vi "总磷总氮通讯.vi"() -> ()   [LabVIEW 2016, in "斯坦道总磷总氮.lvlib"]
uses:
  <vilib>/NI/Modbus Library/API/Wrapper/Create TCP Slave.vi
  <vilib>/Utility/config.llb/Write Key (Boolean).vi
  <vilib>/Utility/config.llb/Write Key (String).vi
  <vilib>/Plasmionique/MB Master/MB_Master/MB_Master.lvclass
  <vilib>/NI/Modbus Library/API/slave/Modbus Slave.lvclass
  <vilib>/Utility/config.llb/NI_LVConfig.lvlib
  <vilib>/Plasmionique/MB Master/MB Master.lvlib
  <vilib>/NI/Modbus Library/API/Wrapper/API Main.lvlib
  <vilib>/ptbypt/NI_PtbyPt.lvlib
panel:
  out "氨氮状态告警区":u16[](array[numeric])
  out "氨氮测量数据区":u16[](array[numeric])
  out "COD测量数据区":u16[](array[numeric])
  out "COD状态告警区":u16[](array[numeric])
  out "总氮测量数据区":u16[](array[numeric])
  out "总氮状态告警区":u16[](array[numeric])
  out "总磷状态告警区":u16[](array[numeric])
  out "总磷测量数据区":u16[](array[numeric])
  out "序列号":string
  out "状态告警区":T1 {"告警代码" items=["无告警", "缺试剂告警", "缺水样告警", "缺蒸馏水告警", "缺标液告警", "仪表漏液告警", "标定异常告警", "超量程告警", "加热异常", "低试剂预警", "超上限告警", "超下限告警", "仪表内部其他异常", "滴定异常告警", "电极异常告警", "量程切换告警", "参数设置告警", "PH电极电位异常", "电导率电极异常", "浊度光度异常", "溶解氧电极异常", "溶解氧光强异常", "温度异常告警", "PH异常告警", "溶解氧异常告警", "电导率异常告警", "浊度异常告警", "叶绿素异常告警", "藻密度异常告警", "蓝绿藻异常告警", "ORP异常告警", "氨氮异常告警", "清洁刷异常告警", "SD卡异常告警", "蓝牙异常告警", "Wifi异常告警", "流程异常告警"]; "故障代码" items=["无故障", "电机故障", "温度故障", "通讯故障", "滴定故障"]}
  out "测量数据区":T2 {"单位" items=["ug/L", "mg/L", "ppm", "mg/m3", "cm", "ppb", "ug/m3", "%", "nmol/mol", "umol/mol", "MPN/L", "MPN/100ml", "ng/m3", "NTU", "无量纲", "ms/cm", "us/cm", "℃", "mV", "万个/L"]}
  out "status":bool
  out "关键参数区":T3
  in  "读关键参数区":bool
  in  "读状态告警区":bool
  in  "读测量数据区":bool
  in  "站号":u16(ring) items=["总磷"=1, "氨氮"=3]
  in  "停止":bool
  in  "启动":bool
  in  "控制命令":u16(ring) items=["启动测量"=1, "标样核查"=2, "零点核查"=3, "跨度核查"=4, "空白测试"=5, "平行样测试"=6, "加标回收"=7, "空白校准"=8, "标样校准"=9, "初始化（清洗）"=10, "停止测试"=11, "仪器重启"=12, "校时"=13, "模式设置"=14, "测量间隔设置"=15]
  in  "控制命令参数":u16[](array[numeric]) format="%04xH"
  in  "VISA Resource":refnum<visa-resource-name>
  in  "启用模块":bool
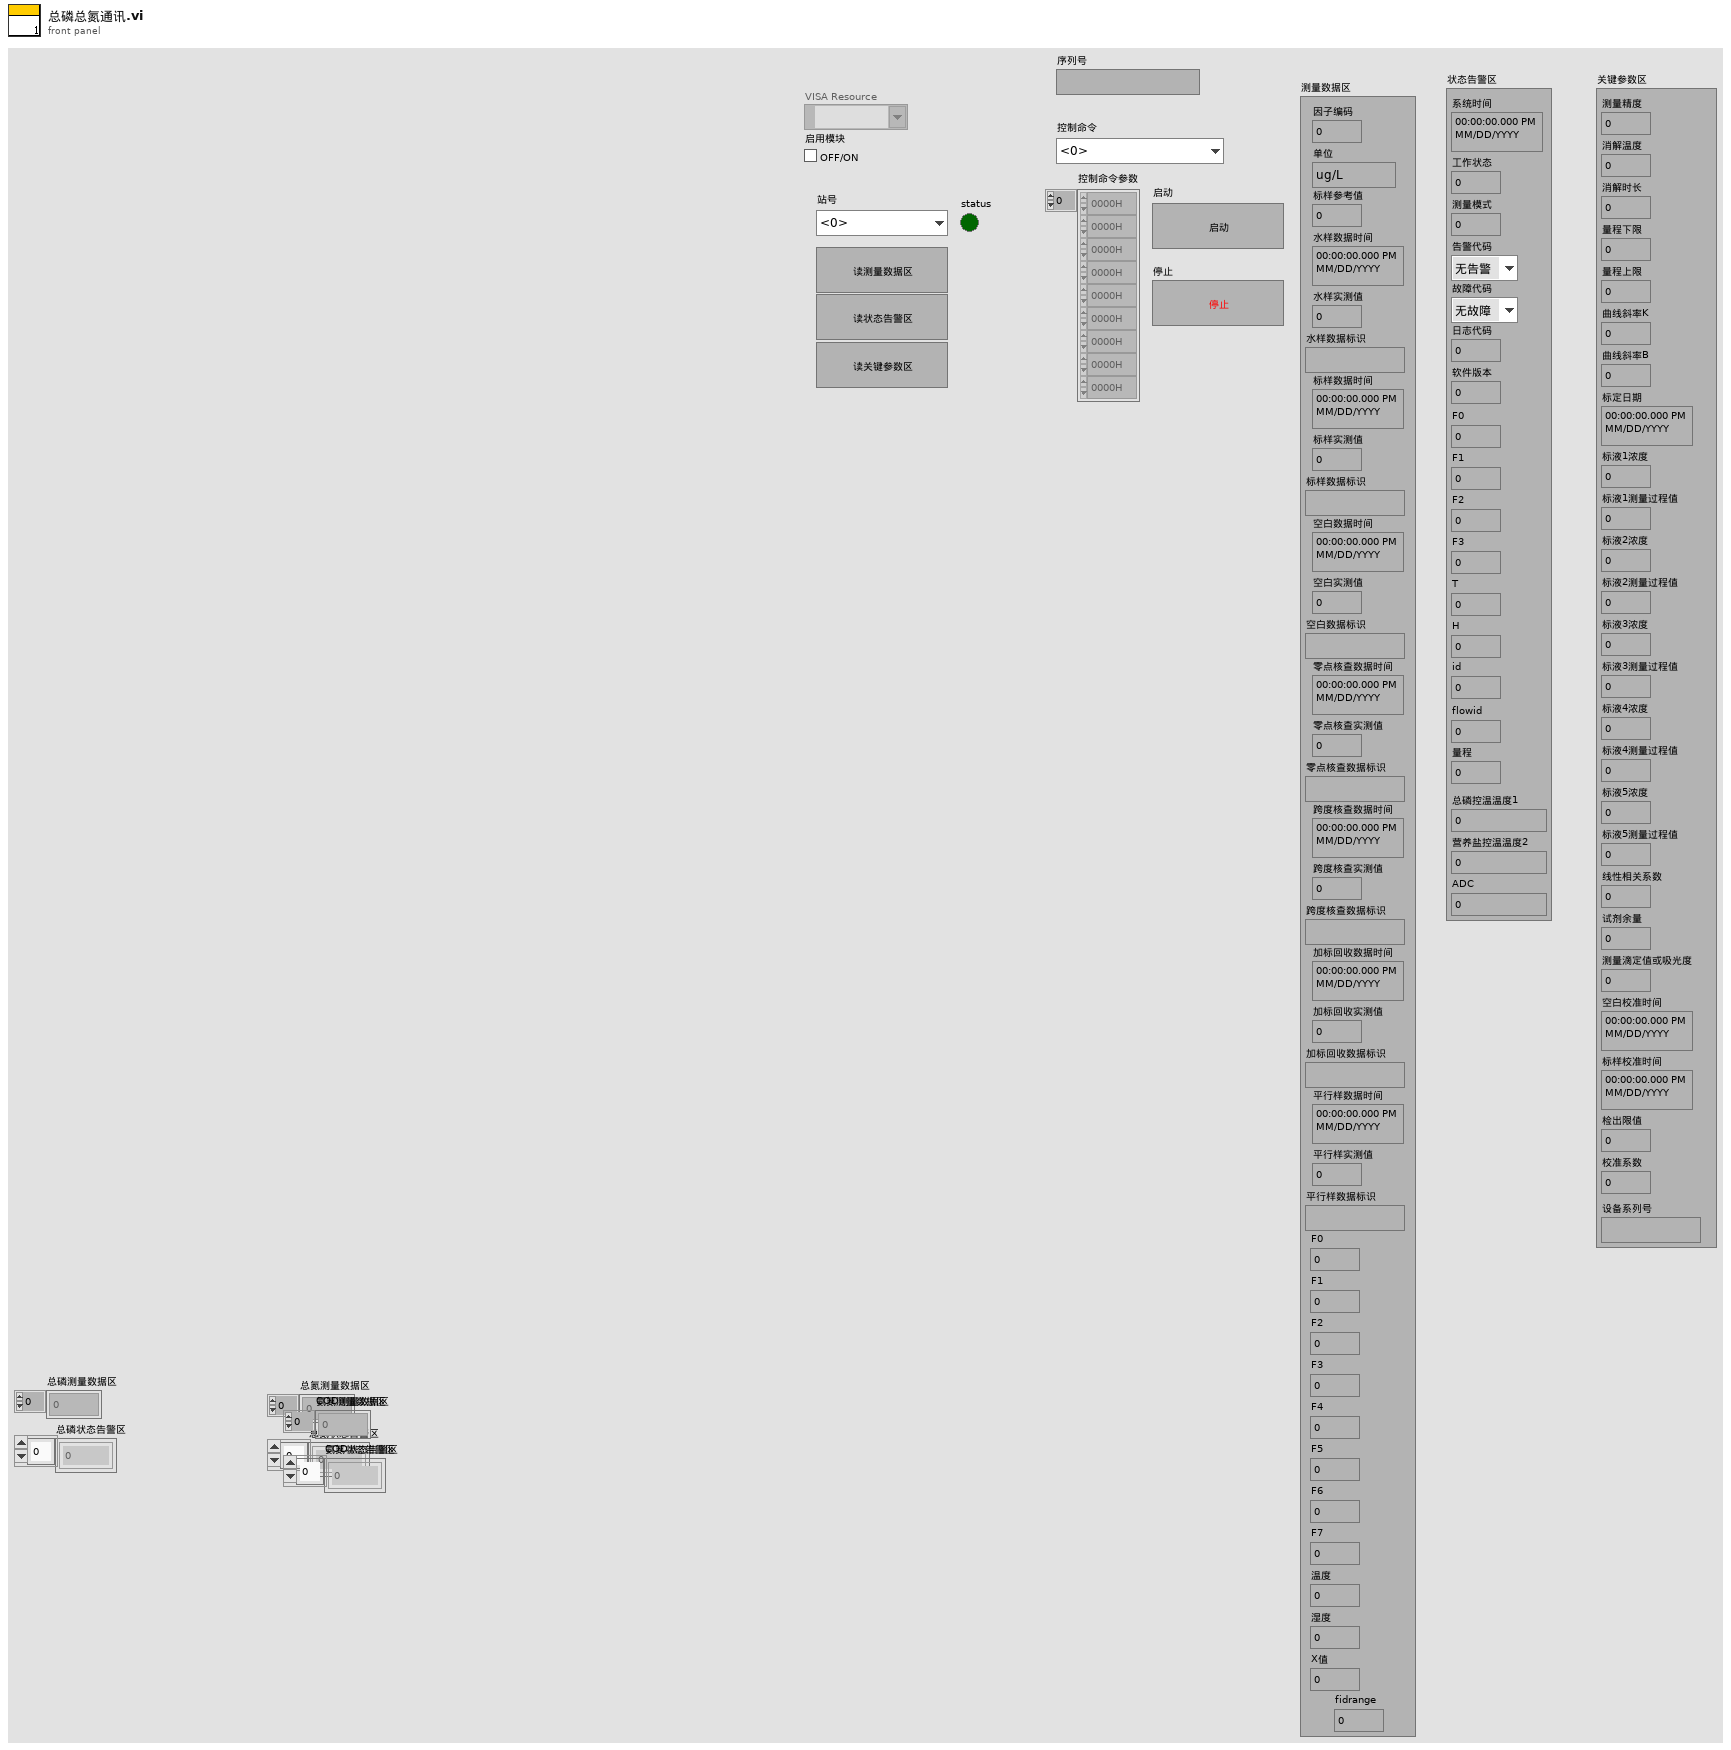
[diagram p1: front panel]
types:
  T1 = cluster{"系统时间":timestamp, "工作状态":u16, "测量模式":u16, "告警代码":u16, "故障代码":u16, "日志代码":u16, "软件版本":u16, "F0":sgl, "F1":sgl, "F2":sgl, "F3":sgl, "T":sgl, "H":sgl, "id":u16, "flowid":u16, "量程":u16, "总磷控温温度1":sgl, "营养盐控温温度2":sgl, "ADC":sgl}
  T2 = cluster{"因子编码":u32, "单位":u16, "标样参考值":sgl, "水样数据时间":timestamp, "水样实测值":sgl, "水样数据标识":string, "标样数据时间":timestamp, "标样实测值":sgl, "标样数据标识":string, "空白数据时间":timestamp, "空白实测值":sgl, "空白数据标识":string, "零点核查数据时间":timestamp, "零点核查实测值":sgl, "零点核查数据标识":string, "跨度核查数据时间":timestamp, "跨度核查实测值":sgl, "跨度核查数据标识":string, "加标回收数据时间":timestamp, "加标回收实测值":sgl, "加标回收数据标识":string, "平行样数据时间":timestamp, "平行样实测值":sgl, "平行样数据标识":string, "F0":sgl, "F1":sgl, "F2":sgl, "F3":sgl, "F4":sgl, "F5":sgl, "F6":sgl, "F7":sgl, "温度":sgl, "湿度":sgl, "X值":sgl, "fidrange":u16}
  T3 = cluster{"测量精度":u16, "消解温度":u16, "消解时长":u16, "量程下限":sgl, "量程上限":sgl, "曲线斜率K":sgl, "曲线斜率B":sgl, "标定日期":timestamp, "标液1浓度":sgl, "标液1测量过程值":sgl, "标液2浓度":sgl, "标液2测量过程值":sgl, "标液3浓度":sgl, "标液3测量过程值":sgl, "标液4浓度":sgl, "标液4测量过程值":sgl, "标液5浓度":sgl, "标液5测量过程值":sgl, "线性相关系数":sgl, "试剂余量":u32, "测量滴定值或吸光度":sgl, "空白校准时间":timestamp, "标样校准时间":timestamp, "检出限值":sgl, "校准系数":sgl, "设备系列号":string}
  T4 = cluster{"COD":bool, "氨氮":bool, "总氮":bool, "总磷":bool}
  T5 = typedef "NI_LVConfig.lvlib/Config Data RefNum.ctl" = refnum<k1>
  T6 = enum8{"Enabled", "Disabled", "Disabled and Grayed Out"}
  T7 = cluster{"时间标识":timestamp, "设备":string, "日志信息":string, "备注":string}
  T8 = cluster{"系统时间":timestamp, "工作状态":enum16{"空闲", "水样测试", "标样核查", "零点核查", "跨度核查", "空白测试", "平行样测试", "加标回收", "空白校准", "标样校准", "初始化（清洗）"}, "测量模式":enum16{"待机", "连续模式", "周期模式", "定点模式", "受控模式", "手动模式"}, "告警代码":u16, "故障代码":u16, "日志代码":u16, "软件版本":u16, "F0":sgl, "F1":sgl, "F2":sgl, "F3":sgl, "T":sgl, "H":sgl, "id":u16, "flowid":u16, "量程":u16, "总磷控温温度1":sgl, "营养盐控温温度2":sgl, "ADC":sgl}
  T9 = cluster{"水样测试量程模式":enum16{"H", "L", "AUTO"}, "空白核查量程模式":enum16{"H", "L", "AUTO"}, "跨度核查量程模式":enum16{"H", "L", "AUTO"}, "加标回收量程模式":enum16{"H", "L", "AUTO"}}
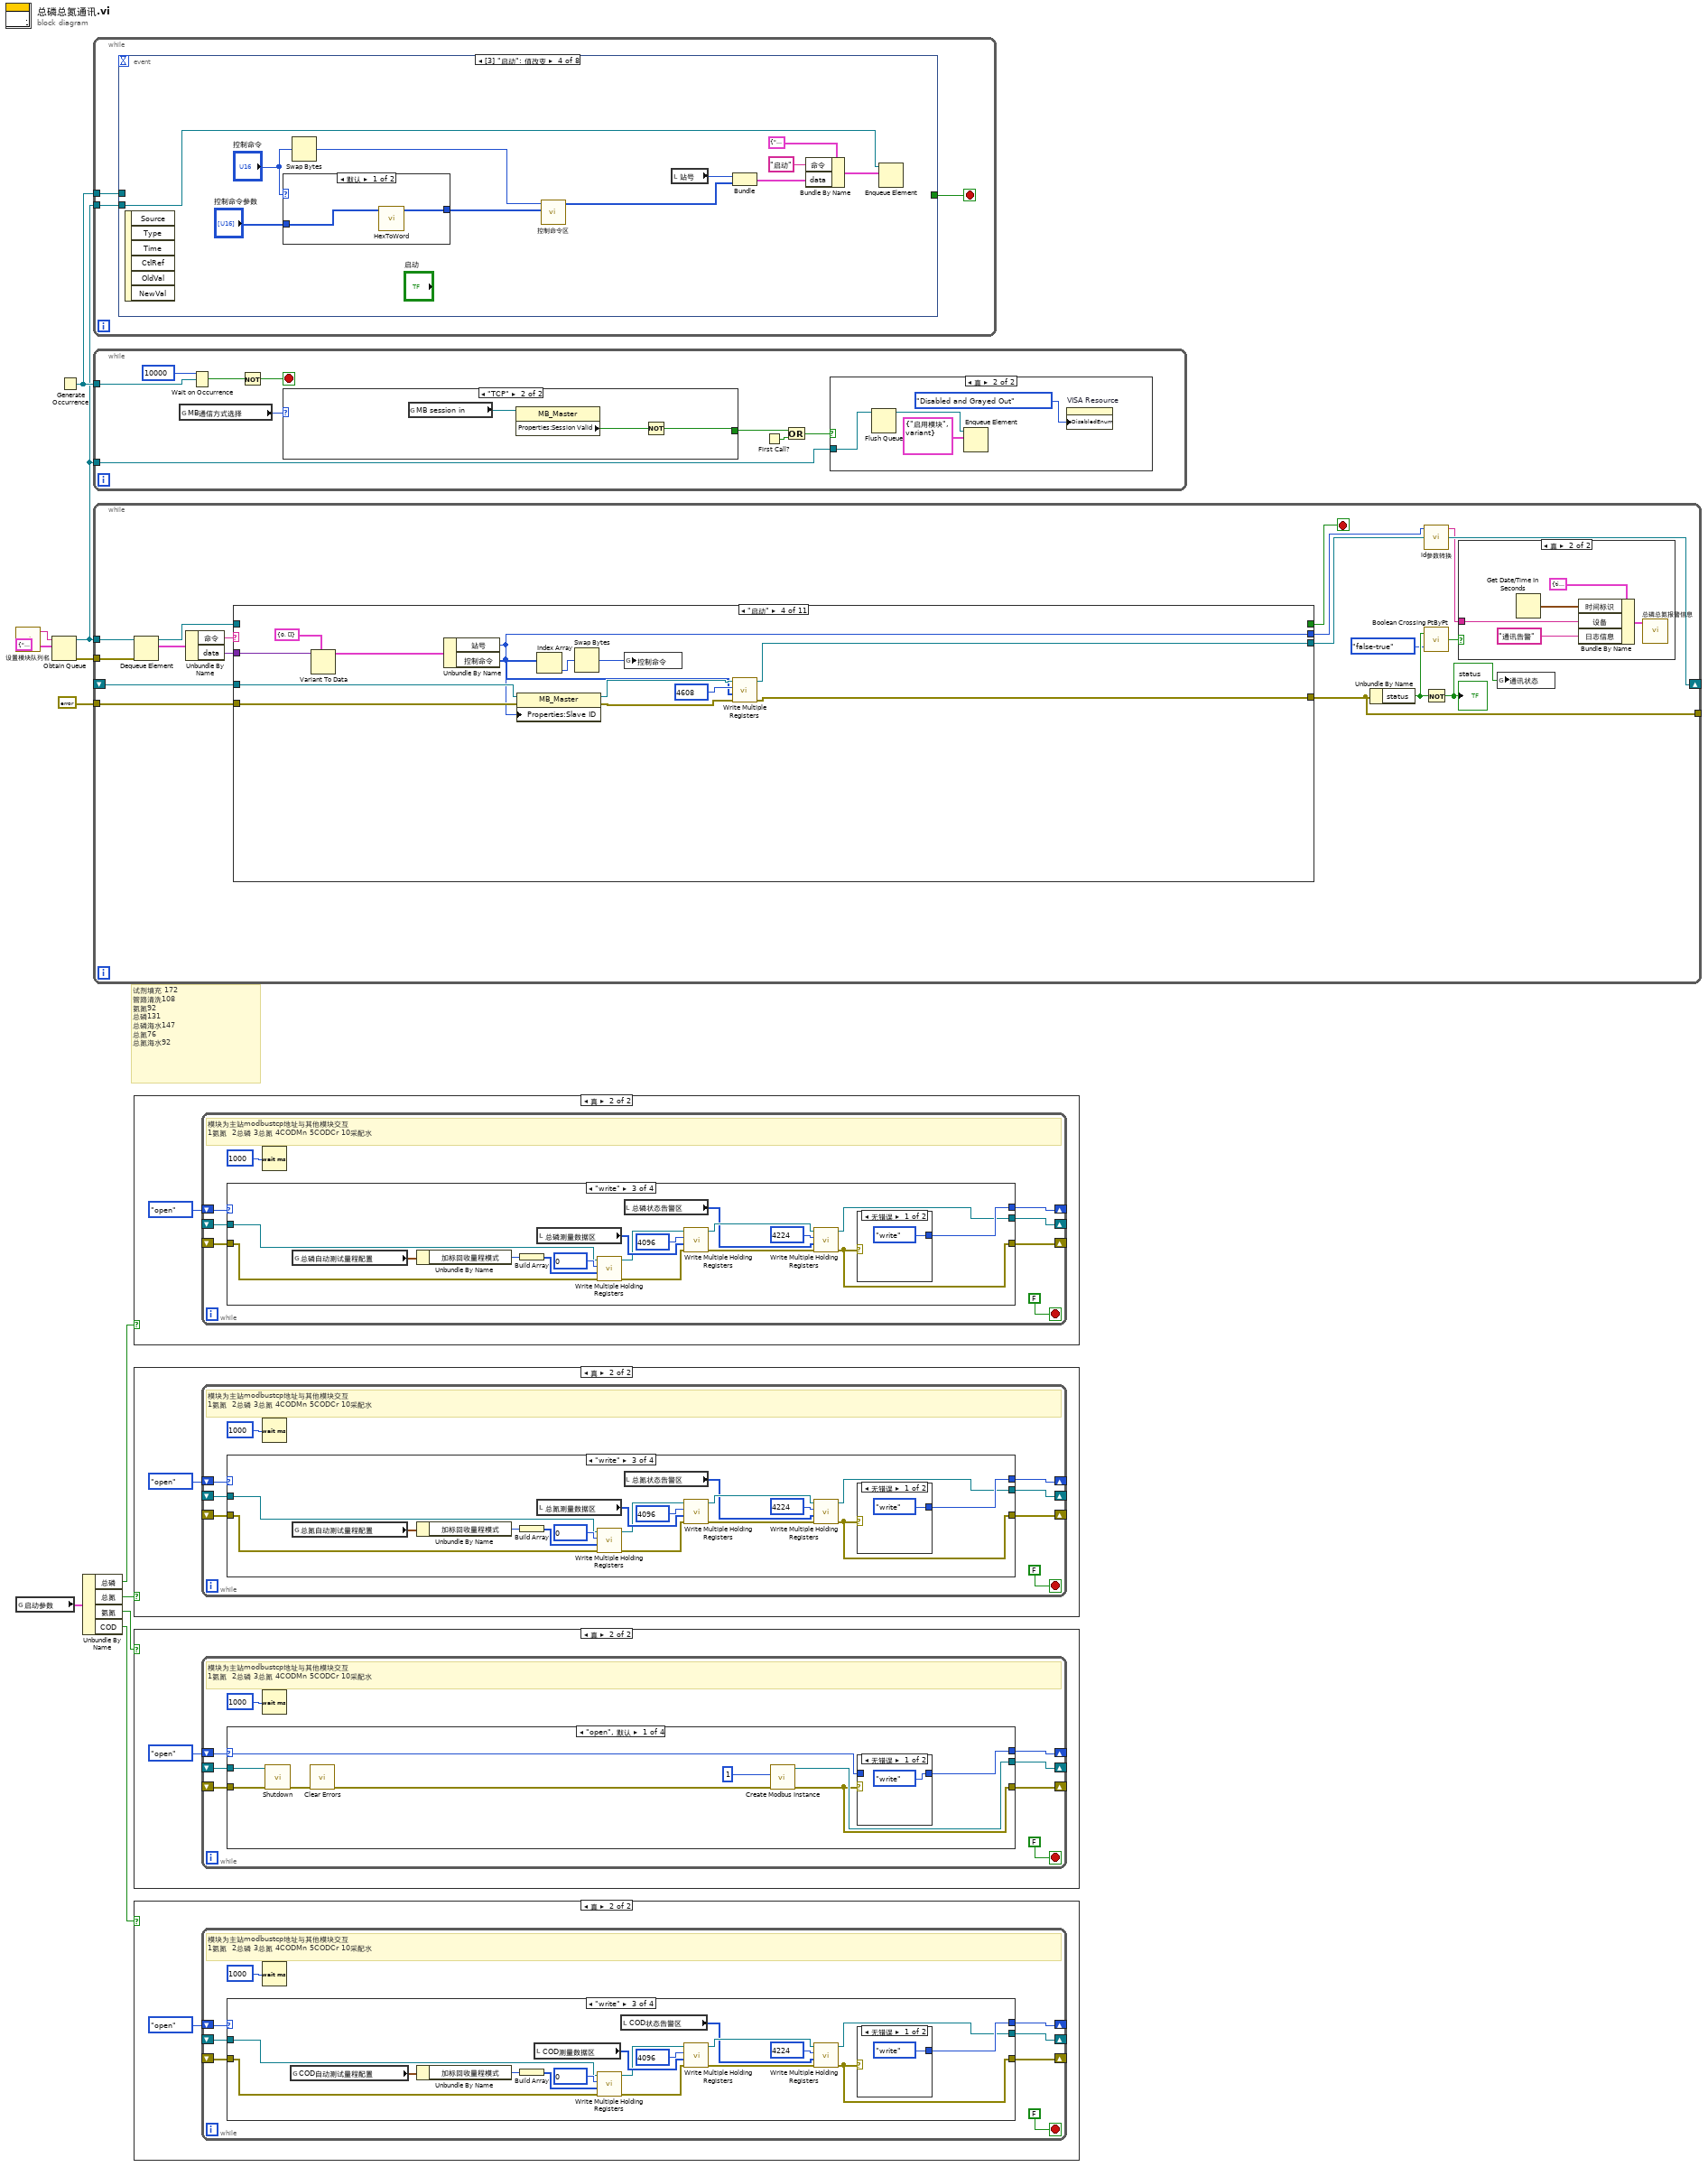
[diagram p0: block diagram]
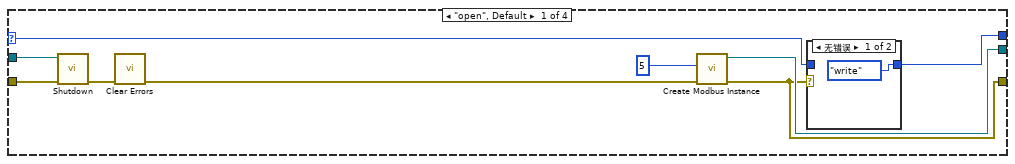
[diagram p3: hidden frame]
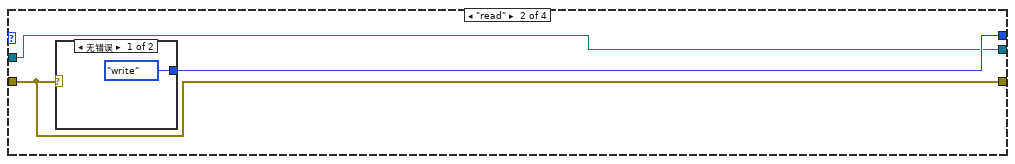
[diagram p5: hidden frame]
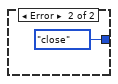
[diagram p6: hidden frame]
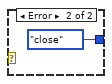
[diagram p7: hidden frame]
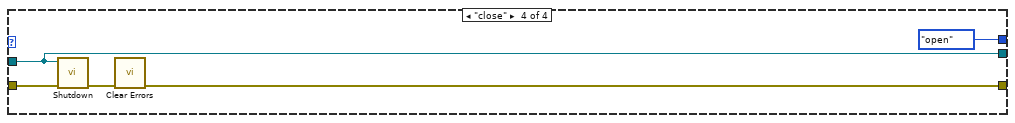
[diagram p8: hidden frame]
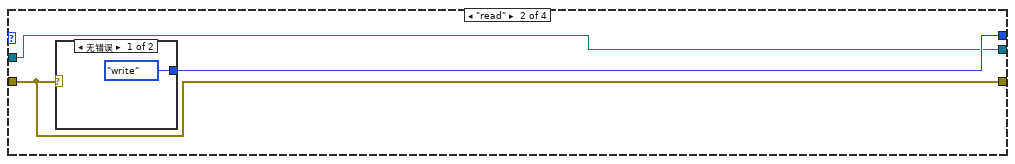
[diagram p11: hidden frame]
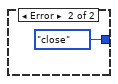
[diagram p12: hidden frame]
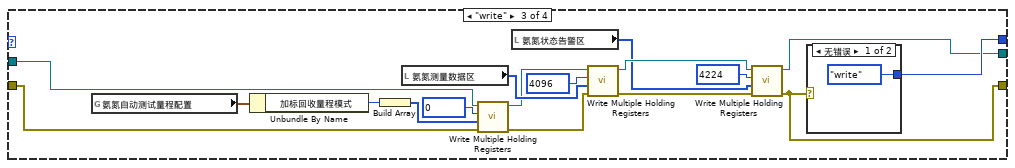
[diagram p13: hidden frame]
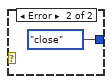
[diagram p14: hidden frame]
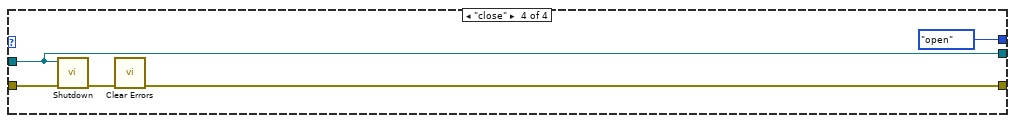
[diagram p15: hidden frame]
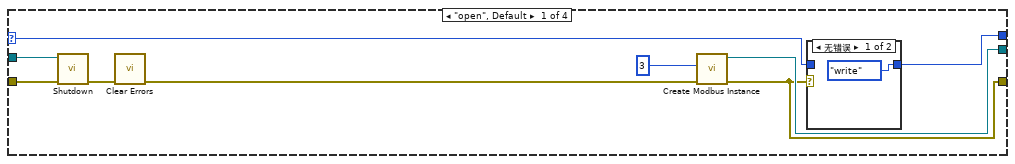
[diagram p17: hidden frame]
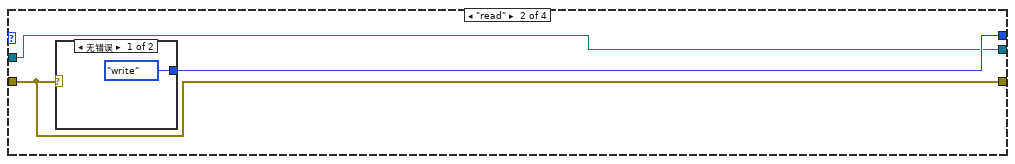
[diagram p19: hidden frame]
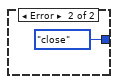
[diagram p20: hidden frame]
diagram:
  # "试剂填充 172 \n管路清洗108\n氨氮92\n总磷131\n总磷海水147\n总氮76\n总氮海水92"
  n1 = call "设置模块队列名.vi"() -> ("Msg"=w1:string)  [unwired: 5 in]
  n2 = global read "总磷总氮断电保存全局变量.vi" "启动参数"() -> (w6:T4)
  n3 = Obtain Queue(name (unnamed)=w1, element data type=cluster{"命令":string, "data":variant} {"命令"="", "data"=variant}) -> (queue out=w7:refnum<queue>, error out=w10:errorcluster)  [unwired: 3 in, 1 out]
  n4 = Generate Occurrence() -> (w8:refnum<k4>)
  n5 = Unbundle By Name(w6) -> ("总磷"=w5:bool, "总氮"=w4:bool, "氨氮"=w3:bool, "COD"=w2:bool)
  n6 = while {
    tunnel: w7 -> [w14]
    tunnel: w8 -> [w12]
    stop <- w13 stop-if-true
    n7 = event shown="[3] \"启动\": 值改变" {
      selector: _ -> [_ _ _ _ _ _ _ _]
      dyn-events: _ -> [_ _ _ _ _ _ _ _]
      timeout: _ -> [_ _ _ _ _ _ _ _]
      tunnel: w14 -> [_ _ _ w45 w52 w58 w63 w68]
      tunnel: [_ _ _ _ "停止" _ _ _] -> w13
      tunnel: w12 -> [_ _ _ _ w49 _ _ _]
      event Timeout {
        n8 = event-data() -> ()  [unwired: 1 in, 3 out]
      }
      event "启用模块": Value Change {
        n9 = event-data() -> ("NewVal"=w15:bool)  [unwired: 1 in, 5 out]
        n10 = call <vilib>:"Application Directory.vi"() -> ("Application Directory"=w17:path)
        n11 = Build Path(base path=w17, name or relative path="data\\set.ini" ("名称或相对路径")) -> (appended path=w18:path)
        n12 = call <vilib>:"Open Config Data.vi"("configuration file path"=w18) -> ("error out"=w24:errorcluster, "refnum"=w23:T5)  [unwired: 8 in, 1 out]
        n13 = call-poly <vilib>:"Write Key.vi"("section"="总磷总氮", "error in (no error)"=w24, "value"=w15, "key"="模块启用", "refnum"=w23) -> ("error out"=w20:errorcluster, "refnum out"=w16:T5)  [unwired: 4 in, 1 out]
        n14 = call <vilib>:"Close Config Data.vi"("error in (no error)"=w20, "refnum"=w16) -> ()  [unwired: 8 in, 2 out]
      }
      event "VISA Resource": Value Change {
        n15 = event-data() -> ()  [unwired: 1 in, 6 out]
        n16 = call <vilib>:"Application Directory.vi"() -> ("Application Directory"=w27:path)
        n17 = Build Path(base path=w27, name or relative path="data\\set.ini" ("名称或相对路径")) -> (appended path=w28:path)
        n18 = call <vilib>:"Open Config Data.vi"("configuration file path"=w28) -> ("error out"=w34:errorcluster, "refnum"=w33:T5)  [unwired: 8 in, 1 out]
        n19 = call-poly <vilib>:"Write Key.vi"("section"="总磷总氮", "error in (no error)"=w34, "value"="VISA Resource", "key"="串口", "refnum"=w33) -> ("error out"=w30:errorcluster, "refnum out"=w26:T5)  [unwired: 4 in, 1 out]
        n20 = call <vilib>:"Close Config Data.vi"("error in (no error)"=w30, "refnum"=w26) -> ()  [unwired: 8 in, 2 out]
      }
      event "启动": Value Change {
        n21 = event-data() -> ()  [unwired: 1 in, 6 out]
        n22 = case shown="默认" "控制命令" {
          tunnel: "控制命令参数" -> [w47 w48]
          tunnel: [w46 w48] -> w35
          frame Default {
            n23 = call "HexToWord.vi"("数组"=w47) -> ("WORD"=w46:u16[])  [unwired: 10 in]
          }
          frame 13 {
          }
        }
        n24 = Swap Bytes(anything="控制命令") -> (byte swapped=w38:u16)
        n25 = call "控制命令区.vi"("控制命令参数"=w35, "控制命令"=w38) -> ("控制命令"=w41:u16[])  [unwired: 9 in]
        n26 = local read "站号"() -> (w40:u16)
        n27 = Bundle("站号"=w40, "控制命令"=w41) -> (w39:cluster{"站号":u16, "控制命令":u16[]})  [unwired: 1 in]
        n28 = Bundle By Name(cluster=cluster{"命令":string, "data":variant} {"命令"="", "data"=variant} ("元素"), "命令"="启动", "data"=w39) -> (w43:cluster{"命令":string, "data":variant})
        n29 = Enqueue Element(queue=w45, element=w43) -> ()  [unwired: 2 in, 3 out]
      }
      event "停止": Value Change {
        n30 = event-data() -> ()  [unwired: 1 in, 6 out]
        n31 = Set Occurrence(w49) -> ()
        n32 = Flush Queue(queue=w52) -> (queue out=w51:refnum<queue>)  [unwired: 1 in, 2 out]
        n33 = Enqueue Element(queue=w51, element=cluster{"命令":string, "data":variant} {"命令"="shutdown", "data"=variant} ("元素")) -> ()  [unwired: 2 in, 3 out]
      }
      event "读测量数据区": Value Change {
        n34 = event-data() -> ()  [unwired: 1 in, 6 out]
        n35 = Bundle By Name(cluster=cluster{"命令":string, "data":variant} {"命令"="", "data"=variant} ("元素"), "命令"="读测量数据区", "data"="站号") -> (w56:cluster{"命令":string, "data":variant})
        n36 = Enqueue Element(queue=w58, element=w56) -> ()  [unwired: 2 in, 3 out]
      }
      event "读状态告警区": Value Change {
        n37 = event-data() -> ()  [unwired: 1 in, 6 out]
        n38 = local read "站号"() -> (w59:u16)
        n39 = Bundle By Name(cluster=cluster{"命令":string, "data":variant} {"命令"="", "data"=variant} ("元素"), "命令"="读状态告警区", "data"=w59) -> (w61:cluster{"命令":string, "data":variant})
        n40 = Enqueue Element(queue=w63, element=w61) -> ()  [unwired: 2 in, 3 out]
      }
      event "读关键参数区": Value Change {
        n41 = event-data() -> ()  [unwired: 1 in, 6 out]
        n42 = local read "站号"() -> (w64:u16)
        n43 = Bundle By Name(cluster=cluster{"命令":string, "data":variant} {"命令"="", "data"=variant} ("元素"), "命令"="读关键参数区", "data"=w64) -> (w66:cluster{"命令":string, "data":variant})
        n44 = Enqueue Element(queue=w68, element=w66) -> ()  [unwired: 2 in, 3 out]
      }
    }
  }
  n45 = while {
    tunnel: w8 -> [w77]
    tunnel: w7 -> [w73]
    stop <- w74 stop-if-true
    n46 = global read "总磷总氮断电保存全局变量.vi" "MB通信方式选择"() -> (w72:enum16{"串口", "TCP"})
    n47 = Wait on Occurrence(2:w77, 3:10000 ("毫秒超时(-1)")) -> (0:w75:bool)  [unwired: 1 in]
    n48 = Not(x=w75) -> (.not. x?=w74:bool)
    n49 = case shown="\"TCP\"" w72 {
      tunnel: [_ w78] -> w69
      frame "串口", Default {
      }
      frame "TCP" {
        n50 = global read "VAR总磷总氮全局变量.vi" "MB session in"() -> (w80:refnum<class "MB_Master.lvclass">)
        n51 = property class="MB_Master"(reference=w80) -> ("Properties:Session Valid"=w79:bool)  [unwired: 1 in, 2 out]
        n52 = Not(x=w79) -> (.not. x?=w78:bool)
      }
    }
    n53 = First Call?() -> (First Call?: T/F=w71:bool)
    n54 = Or(x=w69, y=w71) -> (x .or. y?=w70:bool)
    n55 = case shown="真" w70 {
      tunnel: w73 -> [_ w83]
      frame False {
      }
      frame True {
        n56 = Flush Queue(queue=w83) -> (queue out=w81:refnum<queue>)  [unwired: 1 in, 2 out]
        n57 = Enqueue Element(queue=w81, element=cluster{"命令":string, "data":variant} {"命令"="启用模块", "data"=variant} ("元素")) -> ()  [unwired: 2 in, 3 out]
        n58 = property on="VISA Resource" class="VISAName"("DisabledEnum"=T6."Disabled and Grayed Out" ("禁用")) -> ()  [unwired: 2 in, 2 out]
      }
    }
  }
  n59 = while {
    tunnel: w7 -> [w101]
    tunnel: w10 -> [w100]
    shift-right: [w98] -> _
    shift-left: _ -> [w97]
    tunnel: errorcluster {"status"=FALSE, "code"=0, "source"=""} ("error out") -> [w96]
    tunnel: [w92] -> _
    stop <- w99 stop-if-true
    n60 = Dequeue Element(queue=w101, error in (no error)=w100) -> (queue out=w93:refnum<queue>, element=w94:cluster{"命令":string, "data":variant})  [unwired: 1 in, 2 out]
    n61 = Unbundle By Name(w94) -> ("命令"=w95:string, "data"=w90:variant)
    n62 = case shown="\"启动\"" w95 {
      tunnel: w90 -> [_ _ _ w126 w137 w154 w164 w191 w212 w226 _]
      tunnel: w93 -> [_ _ _ _ _ _ _ _ _ _ w239]
      tunnel: [_ _ _ _ _ _ _ _ _ _ TRUE] -> w99
      tunnel: [w107 w109 w112 w129 w140 w156 w168 w199 w219 w233 w235] -> w98
      tunnel: [w108 w110 w113 w128 w139 w155 w169 w190 w220 w234 w236] -> w92
      tunnel: w97 -> [w107 _ w112 w125 w136 w153 w163 w194 w215 w229 w235]
      tunnel: w96 -> [w108 _ w115 w122 w133 w150 w161 w195 w216 w230 w237]
      tunnel: [_ _ _ w117 w130 w144 w157 w186 w208 w221 _] -> w85
      frame Default {
      }
      frame "启用模块" {
        n63 = call "总磷总氮MB_api.vi"("STEP"=enum16{"open", "read", "write", "close"}."open") -> ("error out"=w110:errorcluster, "MB session out"=w109:refnum<class "MB_Master.lvclass">)  [unwired: 8 in, 1 out]
        n64 = global write "VAR总磷总氮全局变量.vi" "MB session in"(w109) -> ()
      }
      frame "停用模块" {
        n65 = call-dynamic "Close Session.vi"("error in (no error)"=w115, "MB session in"=w112) -> ("error out"=w114:errorcluster)  [unwired: 9 in]
        n66 = call <vilib>:"Clear Errors.vi"("error in (no error)"=w114) -> ("error out"=w113:errorcluster)  [unwired: 5 in, 1 out]
      }
      frame "启动" {
        n67 = Variant To Data(type=cluster{"站号":u16, "控制命令":u16[]} {"站号"=0, "控制命令"=[]} ("输出簇"), Variant=w126) -> (data=w120:cluster{"站号":u16, "控制命令":u16[]})  [unwired: 1 in, 1 out]
        n68 = Unbundle By Name(w120) -> ("站号"=w117:u16, "控制命令"=w118:u16[])
        n69 = property class="MB_Master"(reference=w125, error in=w122, "Properties:Slave ID"=w117) -> (reference out=w124:refnum<class "MB_Master.lvclass">, error out=w123:errorcluster)
        n70 = Index Array(array=w118) -> (element=w119:u16)  [unwired: 1 in]
        n71 = Swap Bytes(anything=w119) -> (byte swapped=w116:u16)
        n72 = global write "VAR总磷总氮全局变量.vi" "控制命令"(w116) -> ()
        n73 = call <vilib>:"Write Multiple Registers.vi"("error in (no error)"=w123, "values"=w118, "starting address"=u16 4608, "MB session in"=w124) -> ("error out"=w128:errorcluster, "MB session out"=w129:refnum<class "MB_Master.lvclass">)  [unwired: 6 in]
      }
      frame "盲样测试" {
        n74 = Variant To Data(type=u8 0, Variant=w137) -> (data=w130:u8)  [unwired: 1 in, 1 out]
        n75 = case shown="默认" w130 {
          tunnel: [u16[] [] ("values") u16[] [33539, 0] ("values") u16[] [23555, 0] ("values")] -> w132
          frame Default {
          }
          frame 1 {
            # "总磷盲样测试命令"
          }
          frame 3 {
            # "氨氮盲样测试"
          }
        }
        n76 = property class="MB_Master"(reference=w136, error in=w133, "Properties:Slave ID"=w130) -> (reference out=w135:refnum<class "MB_Master.lvclass">, error out=w134:errorcluster)
        n77 = call <vilib>:"Write Multiple Registers.vi"("error in (no error)"=w134, "values"=w132, "starting address"=u16 24592, "MB session in"=w135) -> ("error out"=w139:errorcluster, "MB session out"=w140:refnum<class "MB_Master.lvclass">)  [unwired: 6 in]
      }
      frame "debug" {
        n78 = Variant To Data(type=cluster{"站号":u16, "控制命令":u16[]} {"站号"=0, "控制命令"=[]} ("输出簇"), Variant=w154) -> (data=w148:cluster{"站号":u16, "控制命令":u16[]})  [unwired: 1 in, 1 out]
        n79 = Unbundle By Name(w148) -> ("站号"=w144:u16, "控制命令"=w146:u16[])
        n80 = property class="MB_Master"(reference=w153, error in=w150, "Properties:Slave ID"=w144) -> (reference out=w152:refnum<class "MB_Master.lvclass">, error out=w151:errorcluster)
        n81 = Index Array(array=w146) -> (element=w147:u16)  [unwired: 1 in]
        n82 = global write "VAR总磷总氮全局变量.vi" "控制命令"(w147) -> ()
        n83 = call <vilib>:"Write Multiple Registers.vi"("error in (no error)"=w151, "values"=w146, "starting address"=u16 24594, "MB session in"=w152) -> ("error out"=w155:errorcluster, "MB session out"=w156:refnum<class "MB_Master.lvclass">)  [unwired: 6 in]
      }
      frame "读测量数据区" {
        n84 = Variant To Data(type=u8 1 ("Slave ID"), Variant=w164) -> (data=w157:u8)  [unwired: 1 in, 1 out]
        n85 = property class="MB_Master"(reference=w163, error in=w161, "Properties:Slave ID"=w157) -> (reference out=w162:refnum<class "MB_Master.lvclass">, error out=w160:errorcluster)
        n86 = call <vilib>:"Read Holding Registers.vi"("error in (no error)"=w160, "quantity"=u16 105, "starting address"=u16 4096, "MB session in"=w162) -> ("error out"=w169:errorcluster, "Registers"=w158:u16[], "MB session out"=w168:refnum<class "MB_Master.lvclass">)  [unwired: 5 in]
        n87 = call "测量数据区.vi"("数组"=w158) -> ("测量数据区"=w159:T2)  [unwired: 10 in]
        "测量数据区" <- w159
        n88 = global write "VAR总磷总氮全局变量.vi" "测量数据区"(w159) -> ()
        n89 = case shown="3" w157 {
          tunnel: w159 -> [_ w172 w181 w183 w185]
          tunnel: w158 -> [_ w173 w180 w182 w184]
          frame 0, Default {
          }
          frame 1 {
            n90 = global read "总磷总氮断电保存全局变量.vi" "启动参数"() -> (w171:T4)
            n91 = Unbundle By Name(w171) -> ("总氮"=w170:bool)
            n92 = case shown="真" w170 {
              tunnel: [w175 w178] -> w174
              tunnel: w172 -> [w175 w176]
              frame False {
              }
              frame True {
                # "启动总氮时间自动对齐"
                n93 = global read "VAR总磷总氮全局变量.vi" "总磷测量数据区"() -> (w177:T2)
                n94 = global read "VAR总磷总氮全局变量.vi" "总氮测量数据区"() -> (w179:T2)
                n95 = call "总磷数据时间处理.vi"("总磷修正数据输入"=w177, "总氮原始数据"=w179, "总磷原始数据"=w176) -> ("总磷修正数据输出"=w178:T2)  [unwired: 8 in]
              }
            }
            n96 = global write "VAR总磷总氮全局变量.vi" "总磷测量数据区"(w174) -> ()
            "总磷测量数据区" <- w173
          }
          frame 2 {
            n97 = global write "VAR总磷总氮全局变量.vi" "总氮测量数据区"(w181) -> ()
            "总氮测量数据区" <- w180
          }
          frame 3 {
            n98 = global write "VAR总磷总氮全局变量.vi" "氨氮测量数据区"(w183) -> ()
            "氨氮测量数据区" <- w182
          }
          frame 22 {
            n99 = global write "VAR总磷总氮全局变量.vi" "COD测量数据区"(w185) -> ()
            "COD测量数据区" <- w184
          }
        }
      }
      frame "读状态告警区" {
        n100 = Variant To Data(type=u8 1 ("Slave ID"), Variant=w191) -> (data=w186:u8)  [unwired: 1 in, 1 out]
        n101 = property class="MB_Master"(reference=w194, error in=w195, "Properties:Slave ID"=w186) -> (reference out=w193:refnum<class "MB_Master.lvclass">, error out=w192:errorcluster)
        n102 = call <vilib>:"Read Holding Registers.vi"("error in (no error)"=w192, "quantity"=u16 29, "starting address"=u16 4224, "MB session in"=w193) -> ("error out"=w190:errorcluster, "Registers"=w187:u16[], "MB session out"=w199:refnum<class "MB_Master.lvclass">)  [unwired: 5 in]
        n103 = call "状态告警区.vi"("数组"=w187) -> ("状态告警区"=w188:T8)  [unwired: 10 in]
        "状态告警区" <- w188
        n104 = Unbundle By Name(w188) -> ("id"=w189:u16)
        n105 = global write "VAR总磷总氮全局变量.vi" "状态告警区"(w188) -> ()
        n106 = case shown="3" w189 {
          tunnel: w188 -> [_ w201 w203 w205 w207]
          tunnel: w187 -> [_ w200 w202 w204 w206]
          frame 0, Default {
          }
          frame 1, 131 {
            n107 = global write "VAR总磷总氮全局变量.vi" "总磷状态告警区"(w201) -> ()
            "总磷状态告警区" <- w200
          }
          frame 2, 76 {
            n108 = global write "VAR总磷总氮全局变量.vi" "总氮状态告警区"(w203) -> ()
            "总氮状态告警区" <- w202
          }
          frame 3 {
            n109 = global write "VAR总磷总氮全局变量.vi" "氨氮状态告警区"(w205) -> ()
            "氨氮状态告警区" <- w204
          }
          frame 22 {
            n110 = global write "VAR总磷总氮全局变量.vi" "COD状态告警区"(w207) -> ()
            "COD状态告警区" <- w206
          }
        }
      }
      frame "读关键参数区" {
        n111 = Variant To Data(type=u8 1 ("Slave ID"), Variant=w212) -> (data=w208:u8)  [unwired: 1 in, 1 out]
        n112 = property class="MB_Master"(reference=w215, error in=w216, "Properties:Slave ID"=w208) -> (reference out=w214:refnum<class "MB_Master.lvclass">, error out=w213:errorcluster)
        n113 = call <vilib>:"Read Holding Registers.vi"("error in (no error)"=w213, "quantity"=u16 19, "starting address"=u16 4256, "MB session in"=w214) -> ("error out"=w220:errorcluster, "Registers"=w210:u16[], "MB session out"=w219:refnum<class "MB_Master.lvclass">)  [unwired: 5 in]
        n114 = call "关键参数区.vi"("数组"=w210) -> ("关键参数区"=w209:T3)  [unwired: 10 in]
        "关键参数区" <- w209
        n115 = global write "VAR总磷总氮全局变量.vi" "关键参数区"(w209) -> ()
      }
      frame "读序列号" {
        n116 = Variant To Data(type=u8 1 ("Slave ID"), Variant=w226) -> (data=w221:u8)  [unwired: 1 in, 1 out]
        n117 = property class="MB_Master"(reference=w229, error in=w230, "Properties:Slave ID"=w221) -> (reference out=w228:refnum<class "MB_Master.lvclass">, error out=w227:errorcluster)
        n118 = call <vilib>:"Read Holding Registers.vi"("error in (no error)"=w227, "quantity"=u16 6, "starting address"=u16 4, "MB session in"=w228) -> ("error out"=w234:errorcluster, "Registers"=w224:u16[], "MB session out"=w233:refnum<class "MB_Master.lvclass">)  [unwired: 5 in]
        n119 = call "HexToString.vi"("数组"=w224) -> ("STRING"=w223:string[])  [unwired: 10 in]
        n120 = Index Array(array=w223) -> (element=w222:string)  [unwired: 1 in]
        "序列号" <- w222
        n121 = global write "VAR总磷总氮全局变量.vi" "序列号"(w222) -> ()
      }
      frame "shutdown" {
        n122 = call-dynamic "Close Session.vi"("error in (no error)"=w237, "MB session in"=w235) -> ("error out"=w236:errorcluster)  [unwired: 9 in]
        n123 = Flush Queue(queue=w239) -> (queue out=w238:refnum<queue>)  [unwired: 1 in, 2 out]
        n124 = Release Queue(queue=w238) -> ()  [unwired: 2 in, 3 out]
      }
    }
    n125 = Unbundle By Name(w92) -> ("status"=w88:bool)
    n126 = call "id参数转换.vi"("id"=w85) -> ("table输出"=w89:string)  [unwired: 10 in]
    n127 = call <vilib>:"Boolean Crossing PtByPt.vi"("direction"=enum16{"either", "false-true", "true-false"}."false-true", "input"=w88) -> ("crossing"=w87:bool)  [unwired: 1 in]
    n128 = Not(x=w88) -> (.not. x?=w91:bool)
    "status" <- w91
    n129 = case shown="真" w87 {
      tunnel: w89 -> [_ w105]
      frame False {
      }
      frame True {
        n130 = Get Date/Time In Seconds() -> (seconds since 1Jan1904=w104:timestamp)
        n131 = Bundle By Name(cluster=T7 {"时间标识"=timestamp(0 s since 1904-01-01), "设备"="", "日志信息"="", "备注"=""} ("data in"), "时间标识"=w104, "设备"=w105, "日志信息"="通讯告警") -> (w103:T7)
        n132 = call "总磷总氮报警信息.vi"("data in"=w103) -> ()  [unwired: 10 in, 1 out]
      }
    }
    n133 = global write "VAR总磷总氮全局变量.vi" "通讯状态"(w91) -> ()
  }
  n134 = case shown="真" w5 {
    frame False {
    }
    frame True {
      n135 = while {
        shift-right: [w247] -> _
        shift-left: _ -> [w249]
        shift-right: [w246] -> _
        shift-left: _ -> [w248]
        shift-right: [w243] -> _
        shift-left: enum16{"open", "read", "write", "close"}."open" -> [w244]
        stop <- FALSE stop-if-true
        # "模块为主站modbustcp地址与其他模块交互\n1氨氮  2总磷 3总氮 4CODMn 5CODCr 10采配水"
        n136 = case shown="\"write\"" w244 {
          selector: w244 -> [w258 _ _ _]
          tunnel: w249 -> [w252 w261 w272 w287]
          tunnel: w248 -> [w251 w262 w268 w286]
          tunnel: [w255 w261 w278 w287] -> w247
          tunnel: [w254 w262 w277 w289] -> w246
          tunnel: [w257 w263 w282 enum16{"open", "read", "write", "close"}."open"] -> w243
          frame "open", Default {
            n137 = call-dynamic "Shutdown.vi"("error in"=w251, "Modbus slave in"=w252) -> ("error out"=w250:errorcluster)  [unwired: 9 in]
            n138 = call <vilib>:"Clear Errors.vi"("error in (no error)"=w250) -> ("error out"=w253:errorcluster)  [unwired: 5 in, 1 out]
            n139 = call-poly <vilib>:"Create Modbus Instance.vi"("error in"=w253, "port (502)"=u16 2) -> ("error out"=w254:errorcluster, "TCP slave instance"=w255:refnum<class "Modbus Slave.lvclass">)  [unwired: 8 in]
            n140 = case shown="无错误" w254 {
              tunnel: w258 -> [_ w260]
              tunnel: [enum16{"open", "read", "write", "close"}."write" w260] -> w257
              frame No Error {
              }
              frame Error {
              }
            }
          }
          frame "read" {
            n141 = case shown="无错误" w262 {
              tunnel: [enum16{"open", "read", "write", "close"}."write" enum16{"open", "read", "write", "close"}."close"] -> w263
              frame No Error {
              }
              frame Error {
              }
            }
          }
          frame "write" {
            n142 = global read "总磷总氮断电保存全局变量.vi" "总磷自动测试量程配置"() -> (w271:T9)
            n143 = Unbundle By Name(w271) -> ("加标回收量程模式"=w270:enum16{"H", "L", "AUTO"})
            n144 = Build Array(w270) -> (w269:enum16{"H", "L", "AUTO"}[])
            n145 = local read "总磷测量数据区"() -> (w276:u16[])
            n146 = call-dynamic "Write Multiple Holding Registers.vi"("error in"=w268, "registers to write"=w269, "starting address"=u16 0, "Modbus slave in"=w272) -> ("error out"=w266:errorcluster, "Modbus slave out"=w267:refnum<class "Modbus Slave.lvclass">)  [unwired: 6 in]
            n147 = local read "总磷状态告警区"() -> (w274:u16[])
            n148 = call-dynamic "Write Multiple Holding Registers.vi"("error in"=w266, "registers to write"=w276, "starting address"=u16 4096, "Modbus slave in"=w267) -> ("error out"=w279:errorcluster, "Modbus slave out"=w280:refnum<class "Modbus Slave.lvclass">)  [unwired: 6 in]
            n149 = call-dynamic "Write Multiple Holding Registers.vi"("error in"=w279, "registers to write"=w274, "starting address"=u16 4224, "Modbus slave in"=w280) -> ("error out"=w277:errorcluster, "Modbus slave out"=w278:refnum<class "Modbus Slave.lvclass">)  [unwired: 6 in]
            n150 = case shown="无错误" w277 {
              tunnel: [enum16{"open", "read", "write", "close"}."write" enum16{"open", "read", "write", "close"}."close"] -> w282
              frame No Error {
              }
              frame Error {
              }
            }
          }
          frame "close" {
            n151 = call-dynamic "Shutdown.vi"("error in"=w286, "Modbus slave in"=w287) -> ("error out"=w285:errorcluster)  [unwired: 9 in]
            n152 = call <vilib>:"Clear Errors.vi"("error in (no error)"=w285) -> ("error out"=w289:errorcluster)  [unwired: 5 in, 1 out]
          }
        }
        n153 = Wait (ms)(milliseconds to wait=u32 1000 ("等待时间（毫秒）")) -> ()  [unwired: 1 out]
      }
    }
  }
  n154 = case shown="真" w4 {
    frame False {
    }
    frame True {
      n155 = while {
        shift-right: [w296] -> _
        shift-left: _ -> [w298]
        shift-right: [w295] -> _
        shift-left: _ -> [w297]
        shift-right: [w292] -> _
        shift-left: enum16{"open", "read", "write", "close"}."open" -> [w293]
        stop <- FALSE stop-if-true
        # "模块为主站modbustcp地址与其他模块交互\n1氨氮  2总磷 3总氮 4CODMn 5CODCr 10采配水"
        n156 = case shown="\"write\"" w293 {
          selector: w293 -> [w307 _ _ _]
          tunnel: w298 -> [w301 w310 w318 w336]
          tunnel: w297 -> [w300 w311 w317 w335]
          tunnel: [w304 w310 w327 w336] -> w296
          tunnel: [w303 w311 w326 w338] -> w295
          tunnel: [w306 w312 w331 enum16{"open", "read", "write", "close"}."open"] -> w292
          frame "open", Default {
            n157 = call-dynamic "Shutdown.vi"("error in"=w300, "Modbus slave in"=w301) -> ("error out"=w299:errorcluster)  [unwired: 9 in]
            n158 = call <vilib>:"Clear Errors.vi"("error in (no error)"=w299) -> ("error out"=w302:errorcluster)  [unwired: 5 in, 1 out]
            n159 = call-poly <vilib>:"Create Modbus Instance.vi"("error in"=w302, "port (502)"=u16 3) -> ("error out"=w303:errorcluster, "TCP slave instance"=w304:refnum<class "Modbus Slave.lvclass">)  [unwired: 8 in]
            n160 = case shown="无错误" w303 {
              tunnel: w307 -> [_ w309]
              tunnel: [enum16{"open", "read", "write", "close"}."write" w309] -> w306
              frame No Error {
              }
              frame Error {
              }
            }
          }
          frame "read" {
            n161 = case shown="无错误" w311 {
              tunnel: [enum16{"open", "read", "write", "close"}."write" enum16{"open", "read", "write", "close"}."close"] -> w312
              frame No Error {
              }
              frame Error {
              }
            }
          }
          frame "write" {
            n162 = global read "总磷总氮断电保存全局变量.vi" "总氮自动测试量程配置"() -> (w321:T9)
            n163 = Unbundle By Name(w321) -> ("加标回收量程模式"=w320:enum16{"H", "L", "AUTO"})
            n164 = Build Array(w320) -> (w319:enum16{"H", "L", "AUTO"}[])
            n165 = local read "总氮测量数据区"() -> (w325:u16[])
            n166 = call-dynamic "Write Multiple Holding Registers.vi"("error in"=w317, "registers to write"=w319, "starting address"=u16 0, "Modbus slave in"=w318) -> ("error out"=w315:errorcluster, "Modbus slave out"=w316:refnum<class "Modbus Slave.lvclass">)  [unwired: 6 in]
            n167 = local read "总氮状态告警区"() -> (w323:u16[])
            n168 = call-dynamic "Write Multiple Holding Registers.vi"("error in"=w315, "registers to write"=w325, "starting address"=u16 4096, "Modbus slave in"=w316) -> ("error out"=w328:errorcluster, "Modbus slave out"=w329:refnum<class "Modbus Slave.lvclass">)  [unwired: 6 in]
            n169 = call-dynamic "Write Multiple Holding Registers.vi"("error in"=w328, "registers to write"=w323, "starting address"=u16 4224, "Modbus slave in"=w329) -> ("error out"=w326:errorcluster, "Modbus slave out"=w327:refnum<class "Modbus Slave.lvclass">)  [unwired: 6 in]
            n170 = case shown="无错误" w326 {
              tunnel: [enum16{"open", "read", "write", "close"}."write" enum16{"open", "read", "write", "close"}."close"] -> w331
              frame No Error {
              }
              frame Error {
              }
            }
          }
          frame "close" {
            n171 = call-dynamic "Shutdown.vi"("error in"=w335, "Modbus slave in"=w336) -> ("error out"=w334:errorcluster)  [unwired: 9 in]
            n172 = call <vilib>:"Clear Errors.vi"("error in (no error)"=w334) -> ("error out"=w338:errorcluster)  [unwired: 5 in, 1 out]
          }
        }
        n173 = Wait (ms)(milliseconds to wait=u32 1000 ("等待时间（毫秒）")) -> ()  [unwired: 1 out]
      }
    }
  }
  n174 = case shown="真" w3 {
    frame False {
    }
    frame True {
      n175 = while {
        shift-right: [w345] -> _
        shift-left: _ -> [w347]
        shift-right: [w344] -> _
        shift-left: _ -> [w346]
        shift-right: [w341] -> _
        shift-left: enum16{"open", "read", "write", "close"}."open" -> [w342]
        stop <- FALSE stop-if-true
        # "模块为主站modbustcp地址与其他模块交互\n1氨氮  2总磷 3总氮 4CODMn 5CODCr 10采配水"
        n176 = case shown="\"open\", 默认" w342 {
          selector: w342 -> [w356 _ _ _]
          tunnel: w347 -> [w350 w359 w367 w385]
          tunnel: w346 -> [w349 w360 w366 w384]
          tunnel: [w353 w359 w376 w385] -> w345
          tunnel: [w352 w360 w375 w387] -> w344
          tunnel: [w355 w361 w380 enum16{"open", "read", "write", "close"}."open"] -> w341
          frame "open", Default {
            n177 = call-dynamic "Shutdown.vi"("error in"=w349, "Modbus slave in"=w350) -> ("error out"=w348:errorcluster)  [unwired: 9 in]
            n178 = call <vilib>:"Clear Errors.vi"("error in (no error)"=w348) -> ("error out"=w351:errorcluster)  [unwired: 5 in, 1 out]
            n179 = call-poly <vilib>:"Create Modbus Instance.vi"("error in"=w351, "port (502)"=u16 1) -> ("error out"=w352:errorcluster, "TCP slave instance"=w353:refnum<class "Modbus Slave.lvclass">)  [unwired: 8 in]
            n180 = case shown="无错误" w352 {
              tunnel: w356 -> [_ w358]
              tunnel: [enum16{"open", "read", "write", "close"}."write" w358] -> w355
              frame No Error {
              }
              frame Error {
              }
            }
          }
          frame "read" {
            n181 = case shown="无错误" w360 {
              tunnel: [enum16{"open", "read", "write", "close"}."write" enum16{"open", "read", "write", "close"}."close"] -> w361
              frame No Error {
              }
              frame Error {
              }
            }
          }
          frame "write" {
            n182 = global read "总磷总氮断电保存全局变量.vi" "氨氮自动测试量程配置"() -> (w370:T9)
            n183 = Unbundle By Name(w370) -> ("加标回收量程模式"=w369:enum16{"H", "L", "AUTO"})
            n184 = Build Array(w369) -> (w368:enum16{"H", "L", "AUTO"}[])
            n185 = local read "氨氮测量数据区"() -> (w374:u16[])
            n186 = call-dynamic "Write Multiple Holding Registers.vi"("error in"=w366, "registers to write"=w368, "starting address"=u16 0, "Modbus slave in"=w367) -> ("error out"=w364:errorcluster, "Modbus slave out"=w365:refnum<class "Modbus Slave.lvclass">)  [unwired: 6 in]
            n187 = local read "氨氮状态告警区"() -> (w372:u16[])
            n188 = call-dynamic "Write Multiple Holding Registers.vi"("error in"=w364, "registers to write"=w374, "starting address"=u16 4096, "Modbus slave in"=w365) -> ("error out"=w377:errorcluster, "Modbus slave out"=w378:refnum<class "Modbus Slave.lvclass">)  [unwired: 6 in]
            n189 = call-dynamic "Write Multiple Holding Registers.vi"("error in"=w377, "registers to write"=w372, "starting address"=u16 4224, "Modbus slave in"=w378) -> ("error out"=w375:errorcluster, "Modbus slave out"=w376:refnum<class "Modbus Slave.lvclass">)  [unwired: 6 in]
            n190 = case shown="无错误" w375 {
              tunnel: [enum16{"open", "read", "write", "close"}."write" enum16{"open", "read", "write", "close"}."close"] -> w380
              frame No Error {
              }
              frame Error {
              }
            }
          }
          frame "close" {
            n191 = call-dynamic "Shutdown.vi"("error in"=w384, "Modbus slave in"=w385) -> ("error out"=w383:errorcluster)  [unwired: 9 in]
            n192 = call <vilib>:"Clear Errors.vi"("error in (no error)"=w383) -> ("error out"=w387:errorcluster)  [unwired: 5 in, 1 out]
          }
        }
        n193 = Wait (ms)(milliseconds to wait=u32 1000 ("等待时间（毫秒）")) -> ()  [unwired: 1 out]
      }
    }
  }
  n194 = case shown="真" w2 {
    frame False {
    }
    frame True {
      n195 = while {
        shift-right: [w394] -> _
        shift-left: _ -> [w396]
        shift-right: [w393] -> _
        shift-left: _ -> [w395]
        shift-right: [w390] -> _
        shift-left: enum16{"open", "read", "write", "close"}."open" -> [w391]
        stop <- FALSE stop-if-true
        # "模块为主站modbustcp地址与其他模块交互\n1氨氮  2总磷 3总氮 4CODMn 5CODCr 10采配水"
        n196 = case shown="\"write\"" w391 {
          selector: w391 -> [w405 _ _ _]
          tunnel: w396 -> [w399 w408 w416 w434]
          tunnel: w395 -> [w398 w409 w415 w433]
          tunnel: [w402 w408 w425 w434] -> w394
          tunnel: [w401 w409 w424 w436] -> w393
          tunnel: [w404 w410 w429 enum16{"open", "read", "write", "close"}."open"] -> w390
          frame "open", Default {
            n197 = call-dynamic "Shutdown.vi"("error in"=w398, "Modbus slave in"=w399) -> ("error out"=w397:errorcluster)  [unwired: 9 in]
            n198 = call <vilib>:"Clear Errors.vi"("error in (no error)"=w397) -> ("error out"=w400:errorcluster)  [unwired: 5 in, 1 out]
            n199 = call-poly <vilib>:"Create Modbus Instance.vi"("error in"=w400, "port (502)"=u16 5) -> ("error out"=w401:errorcluster, "TCP slave instance"=w402:refnum<class "Modbus Slave.lvclass">)  [unwired: 8 in]
            n200 = case shown="无错误" w401 {
              tunnel: w405 -> [_ w407]
              tunnel: [enum16{"open", "read", "write", "close"}."write" w407] -> w404
              frame No Error {
              }
              frame Error {
              }
            }
          }
          frame "read" {
            n201 = case shown="无错误" w409 {
              tunnel: [enum16{"open", "read", "write", "close"}."write" enum16{"open", "read", "write", "close"}."close"] -> w410
              frame No Error {
              }
              frame Error {
              }
            }
          }
          frame "write" {
            n202 = global read "总磷总氮断电保存全局变量.vi" "COD自动测试量程配置"() -> (w419:T9)
            n203 = Unbundle By Name(w419) -> ("加标回收量程模式"=w418:enum16{"H", "L", "AUTO"})
            n204 = Build Array(w418) -> (w417:enum16{"H", "L", "AUTO"}[])
            n205 = local read "COD测量数据区"() -> (w423:u16[])
            n206 = call-dynamic "Write Multiple Holding Registers.vi"("error in"=w415, "registers to write"=w417, "starting address"=u16 0, "Modbus slave in"=w416) -> ("error out"=w413:errorcluster, "Modbus slave out"=w414:refnum<class "Modbus Slave.lvclass">)  [unwired: 6 in]
            n207 = local read "COD状态告警区"() -> (w421:u16[])
            n208 = call-dynamic "Write Multiple Holding Registers.vi"("error in"=w413, "registers to write"=w423, "starting address"=u16 4096, "Modbus slave in"=w414) -> ("error out"=w426:errorcluster, "Modbus slave out"=w427:refnum<class "Modbus Slave.lvclass">)  [unwired: 6 in]
            n209 = call-dynamic "Write Multiple Holding Registers.vi"("error in"=w426, "registers to write"=w421, "starting address"=u16 4224, "Modbus slave in"=w427) -> ("error out"=w424:errorcluster, "Modbus slave out"=w425:refnum<class "Modbus Slave.lvclass">)  [unwired: 6 in]
            n210 = case shown="无错误" w424 {
              tunnel: [enum16{"open", "read", "write", "close"}."write" enum16{"open", "read", "write", "close"}."close"] -> w429
              frame No Error {
              }
              frame Error {
              }
            }
          }
          frame "close" {
            n211 = call-dynamic "Shutdown.vi"("error in"=w433, "Modbus slave in"=w434) -> ("error out"=w432:errorcluster)  [unwired: 9 in]
            n212 = call <vilib>:"Clear Errors.vi"("error in (no error)"=w432) -> ("error out"=w436:errorcluster)  [unwired: 5 in, 1 out]
          }
        }
        n213 = Wait (ms)(milliseconds to wait=u32 1000 ("等待时间（毫秒）")) -> ()  [unwired: 1 out]
      }
    }
  }
